vi "Close References.vi"(8 "error in (no error)":errorcluster, 10 "Track (File) References":T2, 11 "Refnum in":T1) -> ()   [LabVIEW 2014]
uses:
  Controls/Track (File) References.ctl
  Controls/FPGA Reference.ctl
  <vilib>/FPGAPlugInAG/Dynamic/niLvFpga_Close_Dynamic.vi
  Controls/Application Data.vi
  <vilib>/rvi/interface/nirviCloseFPGA/nirviCloseFPGA.xnode
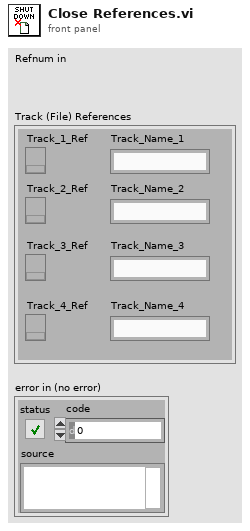
[diagram p1: front panel]
types:
  T1 = typedef "FPGA Reference.ctl" = refnum<k20>
  T2 = typedef "Track (File) References.ctl" = cluster{"Track_1_Ref":refnum<k34>, "Track_2_Ref":refnum<k34>, "Track_3_Ref":refnum<k34>, "Track_4_Ref":refnum<k34>, "Track_Name_1":string, "Track_Name_2":string, "Track_Name_3":string, "Track_Name_4":string}
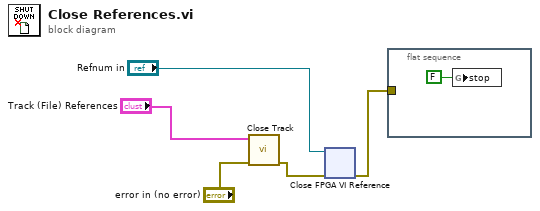
[diagram p0: block diagram]
diagram:
  n1 = call "Close Track.vi"("Error In"="error in (no error)", "Track (File) References"="Track (File) References") -> ("Error Out"=w5:errorcluster)  [unwired: 9 in]
  n2 = xnode "Close FPGA VI Reference"("FPGA VI Reference In"="Refnum in", "error in"=w5) -> ("error out"=w1:errorcluster)
  n3 = flat-sequence {
    tunnel: w1 -> [_]
    frame #0 {
      n4 = global write "Application Data.vi" "stop"(FALSE ("stop")) -> ()
    }
  }
